vi "Configure Modulation (Pulse Width).vi"(0 "VISA resource name":refnum<visa-resource-name>, 1 "Enable Pulse Width Modulation (T: Enable)":bool=TRUE, 2 "File Path":string, 5 "Channel (0: Channel 1)":u16(ring) items=["Channel 1", "Channel 2"], 7 "Pulse Width Modulation Source (0: Internal)":u16(ring) items=["Internal", "External"], 9 "Modulation Waveform (0: Sine)":i32(ring) items=["Sine", "Square", "Triangle", "Ramp", "Down Ramp", "Noise", "User 1", "User 2", "User 3", "User 4", "Edit Memory", "Edit Path"], 11 "error in (no error)":errorcluster, 12 "Modulation Frequency (100.00 Hz)":dbl=100.0, 13 "Peak  Deviation (10 %)":dbl=10.0) -> (4 "VISA resource name out":refnum<visa-resource-name>, 15 "error out":errorcluster)   [LabVIEW 2019, in "Tektronix AFG 3000 Series.lvlib"]
doc: "Configures and enables pulse width modulation. The width of a pulse waveform is varied by the instantaneous voltage of the modulating waveform.\n\n<B>Note:</B>\n\nThe selected waveform must be Pulse which is configured in Configure Standard Waveform.vi for either Channel 1 or Channel 2."
uses:
  Tektronix AFG 3000 Series.lvlib
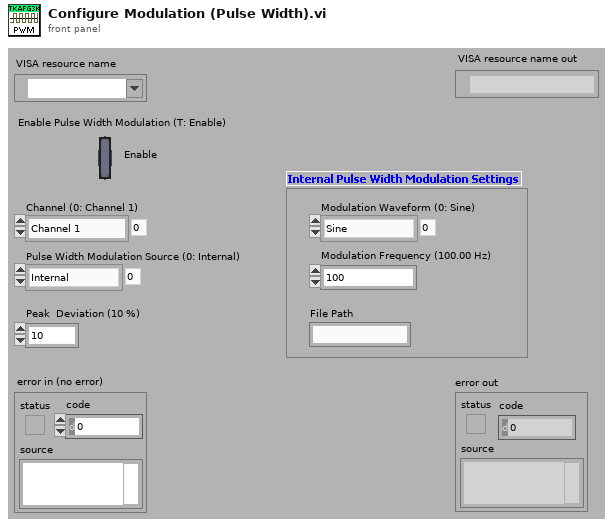
[diagram p1: front panel]
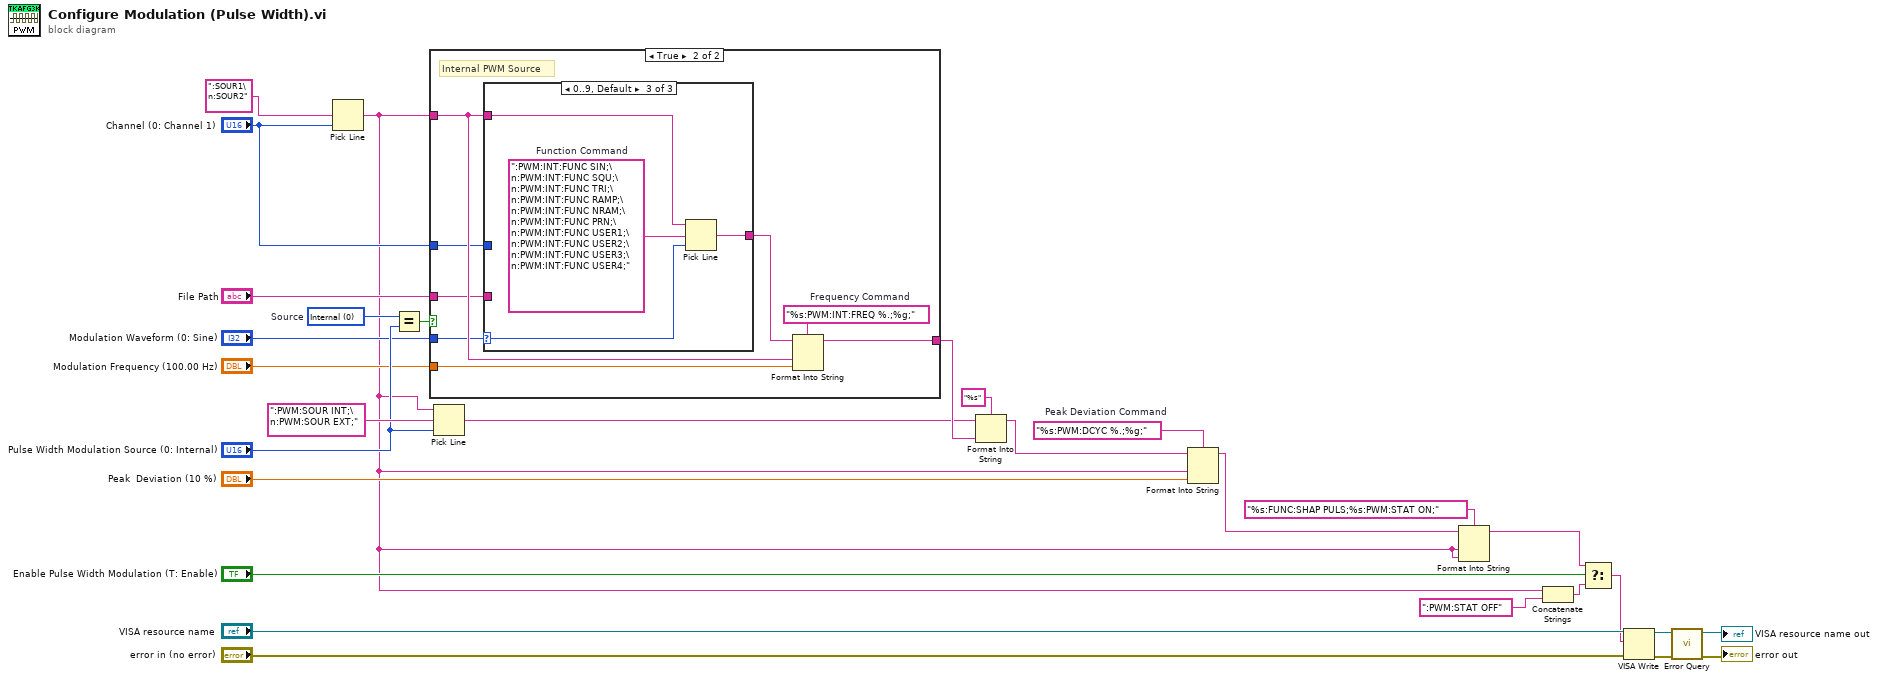
[diagram p0: block diagram]
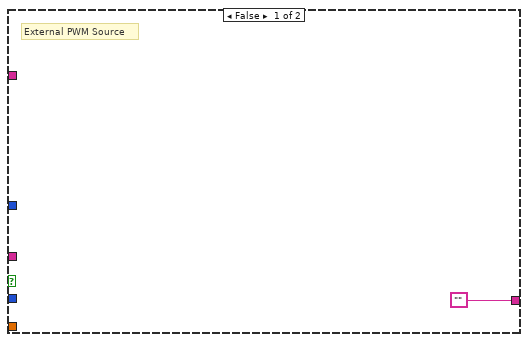
[diagram p2: hidden frame]
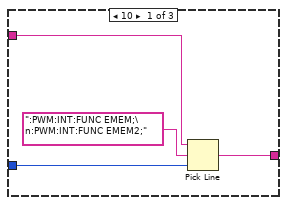
[diagram p3: hidden frame]
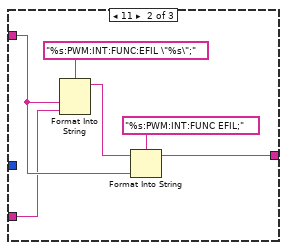
[diagram p4: hidden frame]
diagram:
  w22 = "%s:PWM:DCYC %.;%g;"  # Peak Deviation Command
  w16 = u16 0 items=["Internal", "External"]  # Source
  n1 = Pick Line(multi-line string=":SOUR1\n:SOUR2" ("string (\"\")"), line index="Channel (0: Channel 1)") -> (output string=w2:string)  [unwired: 1 in]
  n2 = Equal?(x=w16, y="Pulse Width Modulation Source (0: Internal)") -> (x = y?=w14:bool)
  n3 = case shown="True" w14 {
    tunnel: ["" w37] -> w12
    tunnel: w2 -> [_ w35]
    tunnel: "Modulation Waveform (0: Sine)" -> [_ w34]
    tunnel: "Modulation Frequency (100.00 Hz)" -> [_ w36]
    tunnel: "File Path" -> [_ w33]
    tunnel: "Channel (0: Channel 1)" -> [_ w31]
    frame False {
      # "External PWM Source"
    }
    frame True {
      w38 = "%s:PWM:INT:FREQ %.;%g;"  # Frequency Command
      # "Internal PWM Source"
      n4 = case shown="0..9, Default" w34 {
        selector: w34 -> [_ _ w50]
        tunnel: w35 -> [w41 w46 w51]
        tunnel: w31 -> [w40 _ _]
        tunnel: w33 -> [_ w45 _]
        tunnel: [w39 w43 w49] -> w32
        frame 10 {
          n5 = Pick Line(string ("")=w41, multi-line string=":PWM:INT:FUNC EMEM;\n:PWM:INT:FUNC EMEM2;", line index=w40) -> (output string=w39:string)
        }
        frame 11 {
          n6 = Format Into String(format string="%s:PWM:INT:FUNC:EFIL \"%s\";", w46, w45) -> (resulting string=w48:string)  [unwired: 2 in, 1 out]
          n7 = Format Into String(format string="%s:PWM:INT:FUNC EFIL;", initial string=w48, w46) -> (resulting string=w43:string)  [unwired: 1 in, 1 out]
        }
        frame 0..9, Default {
          w52 = ":PWM:INT:FUNC SIN;\n:PWM:INT:FUNC SQU;\n:PWM:INT:FUNC TRI;\n:PWM:INT:FUNC RAMP;\n:PWM:INT:FUNC NRAM;\n:PWM:INT:FUNC PRN;\n:PWM:INT:FUNC USER1;\n:PWM:INT:FUNC USER2;\n:PWM:INT:FUNC USER3;\n:PWM:INT:FUNC USER4;"  # Function Command
          n8 = Pick Line(string ("")=w51, multi-line string=w52, line index=w50) -> (output string=w49:string)
        }
      }
      n9 = Format Into String(format string=w38, initial string=w32, w35, w36) -> (resulting string=w37:string)  [unwired: 1 in, 1 out]
    }
  }
  n10 = Pick Line(string ("")=w2, multi-line string=":PWM:SOUR INT;\n:PWM:SOUR EXT;" ("string (\"\")"), line index="Pulse Width Modulation Source (0: Internal)") -> (output string=w11:string)
  n11 = Format Into String(format string="%s", initial string=w11, w12) -> (resulting string=w10:string)  [unwired: 1 in, 1 out]
  n12 = Format Into String(format string=w22, initial string=w10, w2, "Peak  Deviation (10 %)") -> (resulting string=w3:string)  [unwired: 1 in, 1 out]
  n13 = Format Into String(format string="%s:FUNC:SHAP PULS;%s:PWM:STAT ON;", initial string=w3, w2, w2) -> (resulting string=w1:string)  [unwired: 1 in, 1 out]
  n14 = Concatenate Strings(w2, ":PWM:STAT OFF" ("Disable Command")) -> (w18:string)
  n15 = Select(t=w1, s="Enable Pulse Width Modulation (T: Enable)", f=w18) -> (s? t:f=w17:string)
  n16 = VISA Write(VISA resource name="VISA resource name", write buffer=w17, error in (no error)="error in (no error)") -> (VISA resource name out=w28:refnum<visa-resource-name>, error out=w29:errorcluster)  [unwired: 1 out]
  n17 = call "Error Query.vi"("error in (no error)"=w29, "VISA resource name"=w28) -> ("error out"=→"error out":errorcluster, "VISA resource name out"=→"VISA resource name out":refnum<visa-resource-name>)  [unwired: 6 in, 2 out]
